vi "List Timers.vi"(8 "error in (no error)":errorcluster) -> (0 "error out":errorcluster, 2 "Timer Descriptions":string[](array[string]), 3 "Timers":string[](array[string]))   [LabVIEW 2017, in "TimerEngine.lvlib" / "TimerEngine.lvclass"]
uses:
  TimerEngine.lvclass
  TimerEngine.lvclass/TimerEngine.ctl
  _TimerClass/Timer.lvclass/Timer.ctl
  _TimerClass/Timer.lvclass
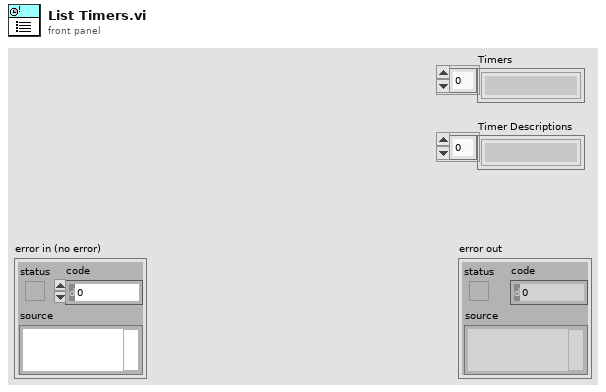
[diagram p1: front panel]
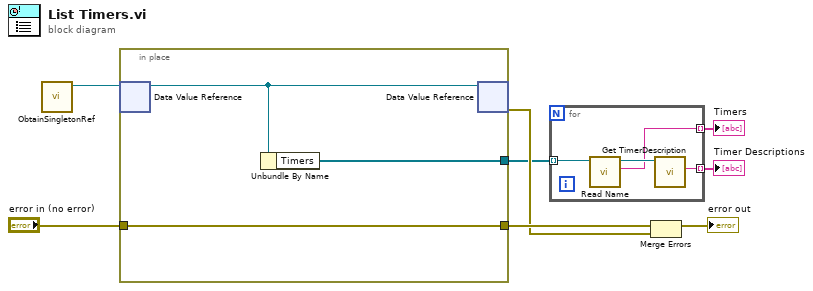
[diagram p0: block diagram]
diagram:
  n1 = call "ObtainSingletonRef.vi"() -> ("data value reference"=w8:refnum<data-value>)  [unwired: 10 in, 1 out]
  n2 = in-place {
    in-place-border: [w11] -> w7
    in-place-border: "error in (no error)" -> [w11]
    in-place-border: [w9] -> w3
    n3 = in-place-dvr #1(w8) -> (w10:refnum<class "TimerEngine.lvclass">)  [unwired: 1 out]
    n4 = Unbundle By Name(w10) -> ("Timers"=w9:refnum<class "Timer.lvclass">[])
    n5 = in-place-dvr #1(w10) -> (w4:errorcluster)  [unwired: 1 out]
  }
  n6 = for {
    tunnel: w3 -> [w15] mode=indexing
    tunnel: [w14] -> w2 mode=indexing
    tunnel: [w12] -> w1 mode=indexing
    n7 = call "Read Name.vi"("Timer in"=w15) -> ("Name"=w12:string, "Timer out"=w13:refnum<class "Timer.lvclass">)  [unwired: 8 in, 1 out]
    n8 = call "Get TimerDescription.vi"("Timer in"=w13) -> ("Timer Description"=w14:string)  [unwired: 8 in, 2 out]
  }
  "Timer Descriptions" <- w2
  "Timers" <- w1
  n9 = Merge Errors(w7, w4) -> (→"error out":errorcluster)
